vi "总磷总氮质控参数设置.vi"(11 "质控参数设置":T2) -> (3 "输出簇":T1)   [LabVIEW 2016, in "斯坦道仪器.lvlib"]
uses:
  <vilib>/Utility/miscctls.llb/LVPointTypeDef.ctl
panel:
  in  "总氮标准液标准浓度":dbl
  in  "总氮跨度标准液浓度":dbl
  in  "总氮零点标准液浓度":dbl
  in  "总氮跨度值":dbl
  in  "取消":bool
  in  "确定":bool
  in  "总磷标准液标准浓度":dbl
  in  "总磷跨度标准液浓度":dbl
  in  "总磷零点标准液浓度":dbl
  in  "总磷跨度值":dbl
  # "质控参数设置"
  # "总氮"
  # "监测参数"
  # "总磷"
  # "跨度值"
  # "零点核查标准液浓度"
  # "跨度核查标准液浓度"
  # "标样核查标准液浓度"
  # "质控参数设置"
  # "总氮"
  # "监测参数"
  # "总磷"
  # "跨度值"
  # "零点核查标准液浓度"
  # "跨度核查标准液浓度"
  # "标样核查标准液浓度"
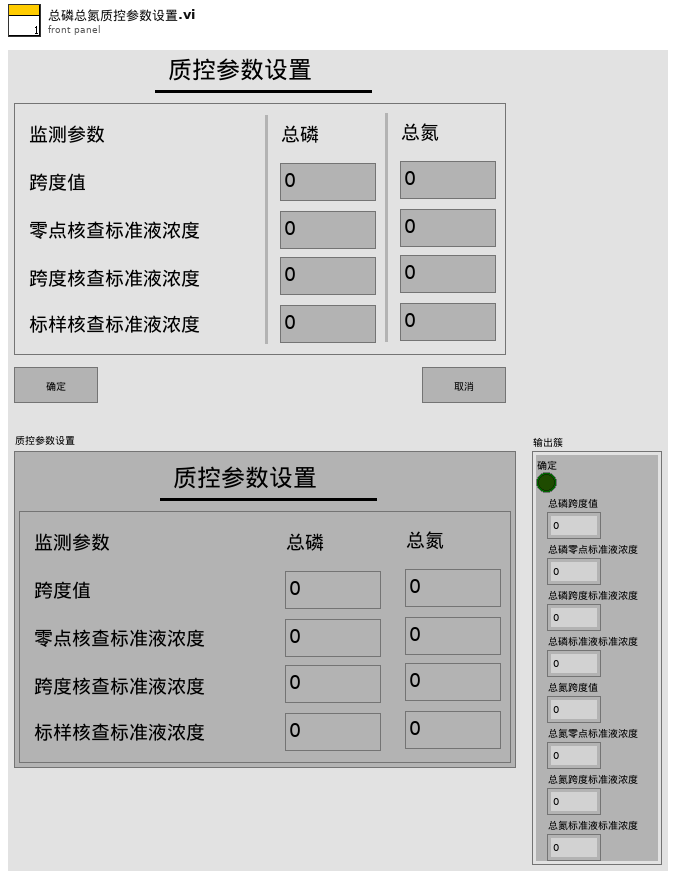
[diagram p1: front panel]
types:
  T1 = cluster{"确定":bool, "总磷跨度值":dbl, "总磷零点标准液浓度":dbl, "总磷跨度标准液浓度":dbl, "总磷标准液标准浓度":dbl, "总氮跨度值":dbl, "总氮零点标准液浓度":dbl, "总氮跨度标准液浓度":dbl, "总氮标准液标准浓度":dbl}
  T2 = cluster{"总磷跨度值":dbl, "总磷零点标准液浓度":dbl, "总磷跨度标准液浓度":dbl, "总磷标准液标准浓度":dbl, "总氮跨度值":dbl, "总氮零点标准液浓度":dbl, "总氮跨度标准液浓度":dbl, "总氮标准液标准浓度":dbl}
  T3 = typedef "LVPointTypeDef.ctl" = cluster{"Horizontal":i16, "Vertical":i16}
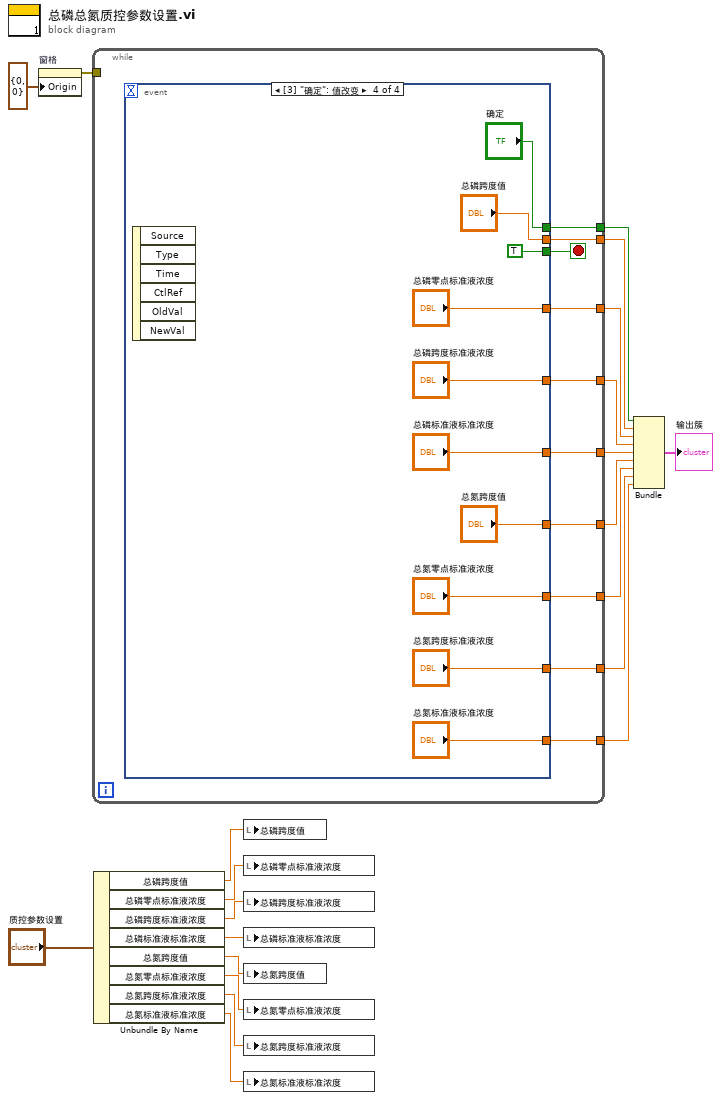
[diagram p0: block diagram]
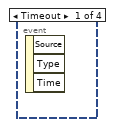
[diagram p2: hidden frame]
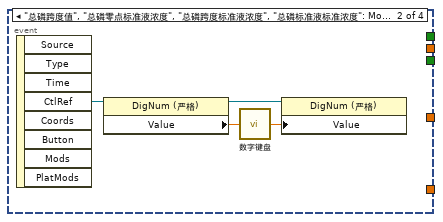
[diagram p3: hidden frame]
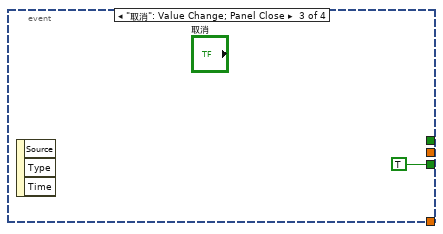
[diagram p4: hidden frame]
diagram:
  n1 = property on="窗格" class="Pane"("Origin"=T3 {"Horizontal"=0, "Vertical"=0} ("原点")) -> (error out=w20:errorcluster)  [unwired: 2 in, 1 out]
  n2 = while {
    tunnel: w20 -> [_]
    tunnel: [w30] -> w19
    tunnel: [w29] -> w18
    tunnel: [w28] -> w17
    tunnel: [w27] -> w16
    tunnel: [w26] -> w15
    tunnel: [w25] -> w5
    tunnel: [w24] -> w4
    tunnel: [w23] -> w3
    tunnel: [w22] -> w2
    stop <- w31 stop-if-true
    n3 = event shown="[3] \"确定\": 值改变" {
      selector: _ -> [_ _ _ _]
      dyn-events: _ -> [_ _ _ _]
      timeout: _ -> [_ _ _ _]
      tunnel: [_ _ TRUE TRUE] -> w31
      tunnel: [_ _ _ "总磷跨度值"] -> w30
      tunnel: [_ _ _ "总磷零点标准液浓度"] -> w29
      tunnel: [_ _ _ "总磷跨度标准液浓度"] -> w28
      tunnel: [_ _ _ "总磷标准液标准浓度"] -> w27
      tunnel: [_ _ _ "确定"] -> w26
      tunnel: [_ _ _ "总氮跨度值"] -> w25
      tunnel: [_ _ _ "总氮零点标准液浓度"] -> w24
      tunnel: [_ _ _ "总氮跨度标准液浓度"] -> w23
      tunnel: [_ _ _ "总氮标准液标准浓度"] -> w22
      event Timeout {
        n4 = event-data() -> ()  [unwired: 1 in, 3 out]
      }
      event "总磷跨度值", "总磷零点标准液浓度", "总磷跨度标准液浓度", "总磷标准液标准浓度": Mouse Down {
        n5 = event-data() -> ("CtlRef"=w35:refnum<vi>)  [unwired: 1 in, 7 out]
        n6 = property class="DigNum (严格)"(reference=w35) -> (reference out=w34:refnum<vi>, "Value"=w33:dbl)  [unwired: 1 in, 1 out]
        n7 = call "数字键盘.vi"("OldNumber"=w33) -> ("NewNumber"=w32:dbl)
        n8 = property class="DigNum (严格)"(reference=w34, "Value"=w32) -> ()  [unwired: 1 in, 2 out]
      }
      event "取消": Value Change; Panel Close {
        n9 = event-data() -> ()  [unwired: 1 in, 3 out]
      }
      event "确定": Value Change {
        n10 = event-data() -> ()  [unwired: 1 in, 6 out]
      }
    }
  }
  n11 = Unbundle By Name("质控参数设置") -> ("总磷跨度值"=w14:dbl, "总磷零点标准液浓度"=w13:dbl, "总磷跨度标准液浓度"=w12:dbl, "总磷标准液标准浓度"=w11:dbl, "总氮跨度值"=w6:dbl, "总氮零点标准液浓度"=w7:dbl, "总氮跨度标准液浓度"=w8:dbl, "总氮标准液标准浓度"=w9:dbl)
  n12 = local write "总磷跨度值"(w14) -> ()
  n13 = local write "总磷零点标准液浓度"(w13) -> ()
  n14 = local write "总磷跨度标准液浓度"(w12) -> ()
  n15 = local write "总磷标准液标准浓度"(w11) -> ()
  n16 = local write "总氮跨度值"(w6) -> ()
  n17 = local write "总氮零点标准液浓度"(w7) -> ()
  n18 = local write "总氮跨度标准液浓度"(w8) -> ()
  n19 = local write "总氮标准液标准浓度"(w9) -> ()
  n20 = Bundle("确定"=w15, "总磷跨度值"=w19, "总磷零点标准液浓度"=w18, "总磷跨度标准液浓度"=w17, "总磷标准液标准浓度"=w16, "总氮跨度值"=w5, "总氮零点标准液浓度"=w4, "总氮跨度标准液浓度"=w3, "总氮标准液标准浓度"=w2) -> (→"输出簇":T1)  [unwired: 1 in]
